vi "SMU Switch Handshaking - LV code improvements - Streaming.vi"(8 "error in":errorcluster, 9 "Error Stream gRPCid":T1, 10 "gRPCid":T1, 11 "file path (use dialog)":path=path "/home/lvuser/jsontestfile.json") -> (0 "error out":errorcluster, 3 "Elapsed Time":u32)   [LabVIEW 2019]
uses:
  VIs/MeasurementServer_gRPCid.ctl
  <instrlib>/niDCPower/nidcpower.llb/niDCPower Send Software Edge Trigger - Signal.ctl
  Global Operations.ctl
  VIs/MeasurementServer_FourProbeRawData.ctl
  VIs/MeasurementServer_ErrorOutData.ctl
  <instrlib>/niDCPower/nidcpower.llb/niDCPower Configure Software Edge Start Trigger.vi
  <instrlib>/niDCPower/nidcpower.llb/niDCPower Configure Software Edge Sequence Advance Trigger.vi
  VIs/labview-grpc-measurement-server.lvlib
  SupportVIs.lvlib
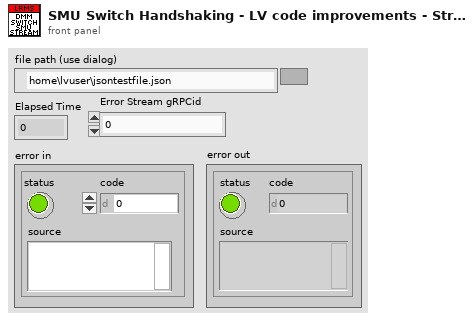
[diagram p1: front panel]
types:
  T1 = typedef "labview-grpc-measurement-server.lvlib/MeasurementServer_gRPCid.ctl" = u64
  T2 = typedef "niDCPower Send Software Edge Trigger - Signal.ctl" = i32
  T3 = typedef "JSONCluster.ctl" = cluster{"SMUResourceName":string, "SMUChannels":string, "SMUSourceMode":i32, "SMUOutputFunction":i32, "SMUSourceTransientResponse":i32, "SMUCurrent":dbl, "SMUCurrentLevelRange":dbl, "SMUMeasurementSense":i32, "SMUMeasurementApertureTime":dbl, "SMUSourceAdvancedSourceDelay":dbl, "SMUVoltage":dbl, "SMUSourceAdvancedSequenceLoopCount":i32, "SMUMeasurementAdvancedDCNoiseRejection":i32, "SMUSequenceName":string, "SMUStep1_Source_DCCurrent_CurrentLevel":i32, "SMUStep2_Measurement_ApertureTime":i32, "SMUStep3_Source_Advanced_SourceDelay":i32, "SMUSequenceNumberOfSteps":i32, "ScanList":string, "Switch1ResourceName":string, "Switch1Topology":string, "Switch1ScanList":string, "Switch2ResourceName":string, "Switch2Topology":string, "Switch2ScanList":string, "DMMResourceName":string, "DMMFunction":i32, "DMMResolution":dbl, "DMMRange":dbl, "DMMSampleCount":i32, "DMMApertureTimeUnit":i32, "DMMApertureTime":dbl, "DMMNumberOfAverages":i32, "DMMAutoZero":i32, "DMMADCCalibration":i32, "DMMSettleTime":dbl, "DMMControlAction":i32, "DMMVoltageFaultUpperLimit":dbl, "ApplicationNumberOfWeldChannels":i32}
  T4 = typedef "Global Operations.ctl" = enum16{"Get", "Set"}
  T5 = typedef "labview-grpc-measurement-server.lvlib/MeasurementServer_ErrorOutData.ctl" = cluster{"ErrorCode":i32, "ErrorMessage":string}
  T6 = typedef "labview-grpc-measurement-server.lvlib/MeasurementServer_FourProbeRawData.ctl" = cluster{"Positive Voltage":dbl, "Positive Current":dbl, "Negative Voltage":dbl, "Negative Current":dbl, "Impedance":dbl, "ErrorOutData":T5}
  T7 = typedef "niDMM Acquisition State.ctl" = enum16{"Running", "Finished with Backlog", "Finished with no Backlog", "Paused", "No acquisition in progress"}
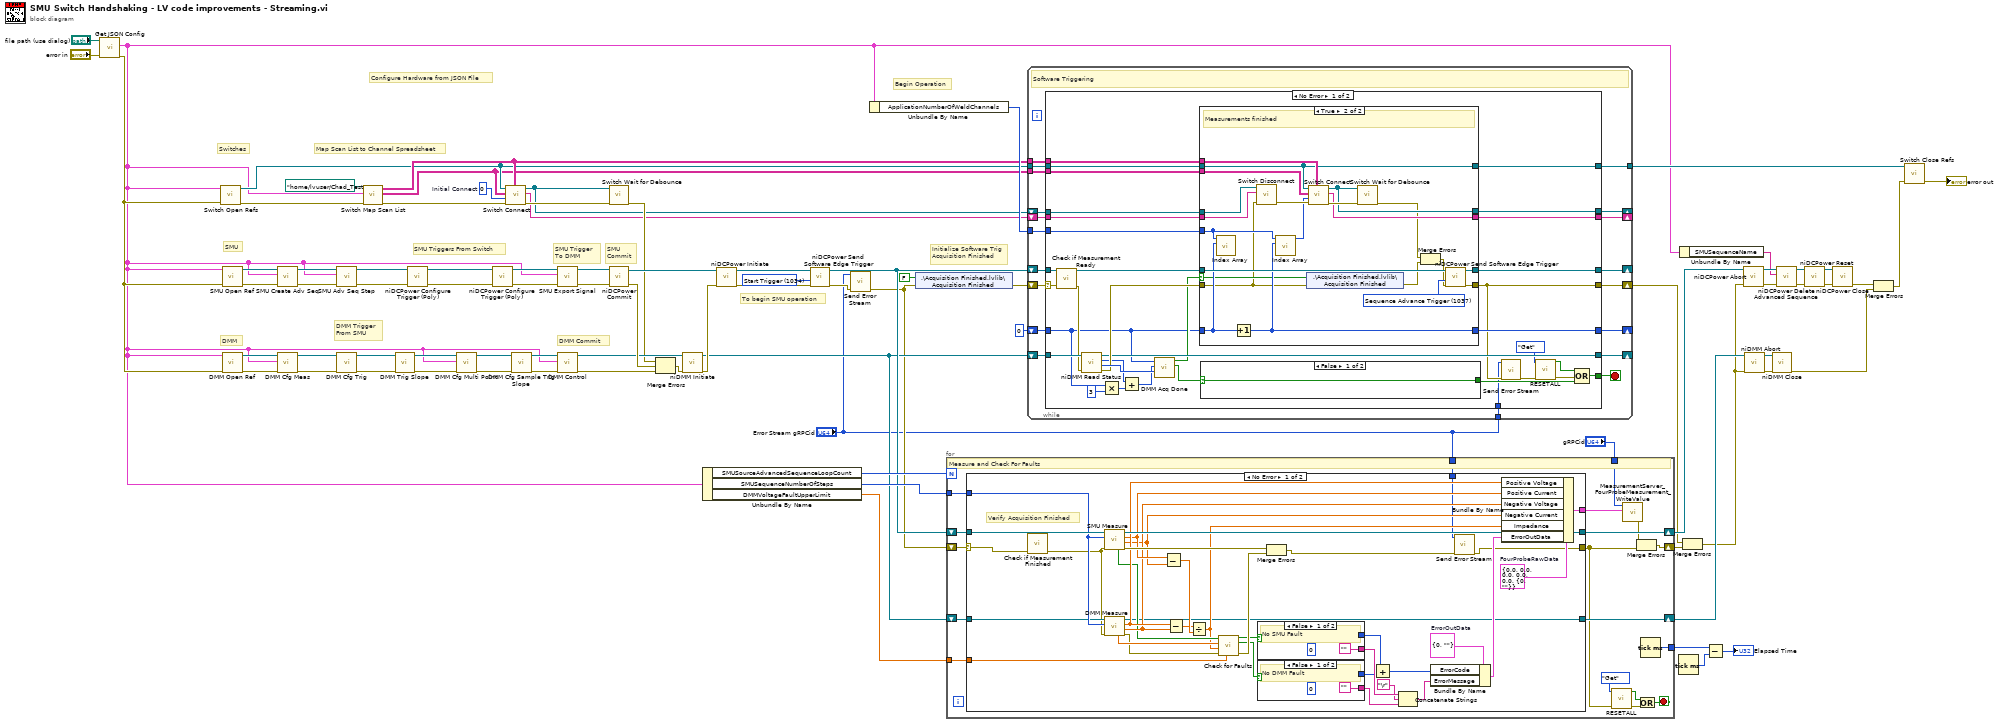
[diagram p0: block diagram]
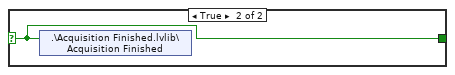
[diagram p2: hidden frame]
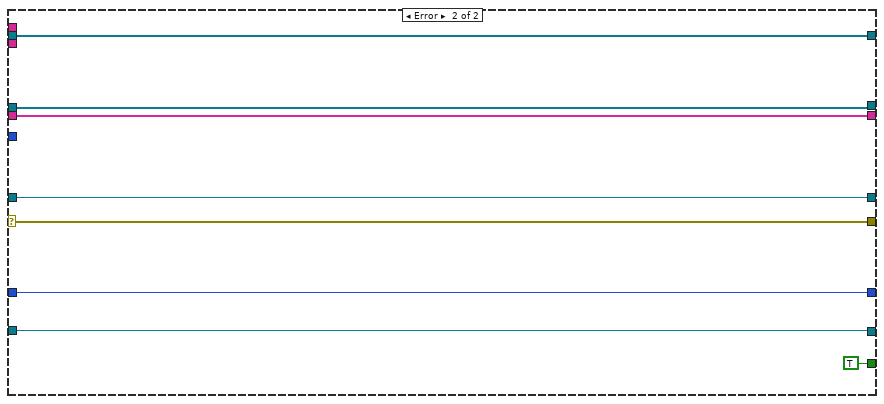
[diagram p4: hidden frame]
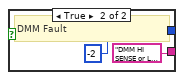
[diagram p5: hidden frame]
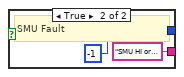
[diagram p6: hidden frame]
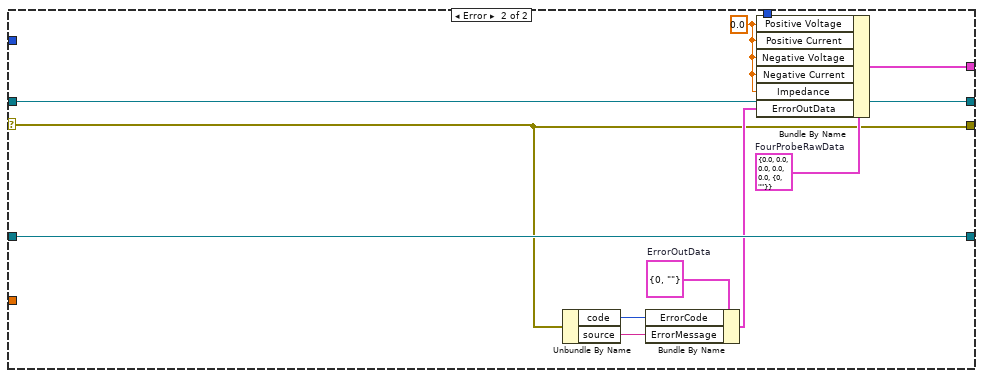
[diagram p7: hidden frame]
diagram:
  w12 = 0  # Initial Connect
  w35 = T2 1034 items=["Start Trigger"=1034, "Source Trigger"=1035, "Measure Trigger"=1036, "Sequence Advance Trigger"=1037, "Pulse Trigger"=1053] ("signal")
  # "Map Scan List to Channel Spreadsheet"
  # "Initialize Software Trig\nAcquisition Finished"
  # "SMU\nCommit"
  # "DMM Commit"
  # "Begin Operation"
  # "Configure Hardware from JSON File"
  # "DMM"
  # "SMU"
  # "Switches"
  # "To begin SMU operation"
  # "DMM Trigger\nFrom SMU"
  # "SMU Trigger \nTo DMM"
  # "SMU Triggers From Switch"
  n1 = call "Get JSON Config.vi"("error in (no error)"="error in", "JSON Configuration File (.json)"="file path (use dialog)") -> ("error out"=w11:errorcluster, "JSONCluster"=w1:T3)  [unwired: 6 in, 2 out]
  n2 = call "Switch Open Refs.vi"("error in (no error)"=w11, "JSONCluster"=w1) -> ("error out"=w15:errorcluster, "Switch Refs"=w8:refnum<k15>[])  [unwired: 8 in]
  n3 = call "SMU Open Ref.vi"("error in (no error)"=w11, "JSONCluster"=w1) -> ("error out"=w82:errorcluster, "IVI Refnum out"=w83:refnum<k15>)  [unwired: 8 in]
  n4 = call "DMM Open Ref.vi"("error in"=w11, "JSONCluster"=w1) -> ("error out"=w55:errorcluster, "IVI Refnum out"=w54:refnum<k15>)  [unwired: 8 in]
  n5 = call "SMU Create Adv Seq.vi"("error in (no error)"=w82, "JSONCluster"=w1, "IVI Refnum in"=w83) -> ("error out"=w70:errorcluster, "IVI Refnum out"=w71:refnum<k15>)  [unwired: 7 in]
  n6 = call "DMM Cfg Meas.vi"("error in (no error)"=w55, "JSONCluster"=w1, "IVI Refnum in"=w54) -> ("error out"=w59:errorcluster, "IVI Refnum out"=w58:refnum<k15>)  [unwired: 7 in]
  n7 = call "SMU Adv Seq Step.vi"("error in (no error)"=w70, "JSONCluster"=w1, "IVI Refnum in"=w71) -> ("error out"=w68:errorcluster, "IVI Refnum out"=w69:refnum<k15>)  [unwired: 7 in]
  n8 = call "DMM Cfg Trig.vi"("error in (no error)"=w59, "IVI Refnum in"=w58) -> ("error out"=w61:errorcluster, "IVI Refnum out"=w60:refnum<k15>)  [unwired: 8 in]
  n9 = call "Switch Map Scan List.vi"("error in (no error)"=w15, "JSONCluster"=w1, "Ch Spreadsheet"=path "/home/lvuser/Chad_Test.csv") -> ("error out"=w14:errorcluster, "IVI Specifications"=w7:string[][], "Channel Specs"=w9:string[][])  [unwired: 6 in]
  n10 = call "DMM Trig Slope.vi"("error in (no error)"=w61, "IVI Refnum in"=w60) -> ("error out"=w63:errorcluster, "IVI Refnum out"=w62:refnum<k15>)  [unwired: 8 in]
  n11 = call-poly <instrlib>:"niDCPower Configure Trigger (Poly).vi"("error in (no error)"=w68, "instrument handle"=w69) -> ("error out"=w79:errorcluster, "instrument handle out"=w80:refnum<k15>)  [unwired: 8 in]
  n12 = call "DMM Cfg Multi Point.vi"("error in (no error)"=w63, "JSONCluster"=w1, "IVI Refnum in"=w62) -> ("error out"=w65:errorcluster, "IVI Refnum out"=w64:refnum<k15>)  [unwired: 7 in]
  n13 = call-poly <instrlib>:"niDCPower Configure Trigger (Poly).vi"("error in (no error)"=w79, "instrument handle"=w80) -> ("error out"=w42:errorcluster, "instrument handle out"=w43:refnum<k15>)  [unwired: 8 in]
  n14 = call "Switch Connect.vi"("Channel Specs"=w9, "error in (no error)"=w14, "Channel Index"=w12, "IVI Specifications"=w7, "Switch Refs"=w8) -> ("error out"=w13:errorcluster, "Channels Connected"=w5:string[], "Refs Connected"=w6:refnum<k15>[])  [unwired: 4 in]
  n15 = call "DMM Cfg Sample Trig Slope.vi"("error in (no error)"=w65, "IVI Refnum in"=w64) -> ("error out"=w47:errorcluster, "IVI Refnum out"=w48:refnum<k15>)  [unwired: 8 in]
  n16 = call "SMU Export Signal.vi"("error in (no error)"=w42, "JSONCluster"=w1, "IVI Refnum in"=w43) -> ("error out"=w66:errorcluster, "IVI Refnum out"=w67:refnum<k15>)  [unwired: 7 in]
  n17 = call "DMM Control.vi"("error in (no error)"=w47, "JSONCluster"=w1, "IVI Refnum in"=w48) -> ("error out"=w52:errorcluster, "IVI Refnum out"=w49:refnum<k15>)  [unwired: 7 in]
  n18 = call "Switch Wait for Debounce.vi"("error in (no error)"=w13, "Switch Refs"=w6) -> ("error out"=w10:errorcluster)  [unwired: 9 in]
  n19 = call <instrlib>:"niDCPower Commit.vi"("error in (no error)"=w66, "instrument handle"=w67) -> ("error out"=w53:errorcluster, "instrument handle out"=w50:refnum<k15>)  [unwired: 8 in]
  n20 = Merge Errors(w10, w53, w52) -> (w51:errorcluster)
  n21 = call <instrlib>:"niDMM Initiate.vi"("error in (no error)"=w51, "instrument handle"=w49) -> ("error out"=w31:errorcluster, "instrument handle out"=w26:refnum<k15>)  [unwired: 8 in]
  n22 = Unbundle By Name(w1) -> ("SMUSourceAdvancedSequenceLoopCount"=w38:i32, "SMUSequenceNumberOfSteps"=w37:i32, "DMMVoltageFaultUpperLimit"=w22:dbl)
  n23 = call <instrlib>:"niDCPower Initiate.vi"("error in (no error)"=w31, "instrument handle"=w50) -> ("error out"=w32:errorcluster, "instrument handle out"=w36:refnum<k15>)  [unwired: 8 in]
  n24 = call <instrlib>:"niDCPower Send Software Edge Trigger.vi"("error in (no error)"=w32, "signal"=w35, "instrument handle"=w36) -> ("error out"=w19:errorcluster, "instrument handle out"=w27:refnum<k15>)  [unwired: 7 in]
  n25 = call "Send Error Stream.vi"("error in (no error)"=w19, "Error Stream gRPCid"="Error Stream gRPCid") -> ("error out"=w18:errorcluster)  [unwired: 9 in]
  n26 = Unbundle By Name(w1) -> ("ApplicationNumberOfWeldChannels"=w33:i32)
  n27 = shared-variable ".\\Acquisition Finished.lvlib\\Acquisition Finished"(FALSE ("Measurement Finished"), error in=w18) -> (error out=w24:errorcluster)
  n28 = for {
    N: w38 -> [_]
    tunnel: w37 -> [w96]
    shift-right: [w94] -> w28
    shift-left: w18 -> [w85]
    shift-right: [w101] -> w81
    shift-left: w27 -> [w97]
    shift-right: [w92] -> w44
    shift-left: w26 -> [w93]
    tunnel: [w100] -> w29
    tunnel: "gRPCid" -> [w99]
    tunnel: w22 -> [w91]
    tunnel: "Error Stream gRPCid" -> [w84]
    stop <- w86 stop-if-true
    # "Measure and Check For Faults"
    n29 = case shown="No Error" w85 {
      selector: w85 -> [w105 w147]
      tunnel: [w137 w155] -> w101
      tunnel: [w113 w148] -> w98
      tunnel: w97 -> [w112 w155]
      tunnel: w96 -> [w111 _]
      tunnel: w93 -> [w110 w154]
      tunnel: [w108 w154] -> w92
      tunnel: w91 -> [w106 _]
      tunnel: [w103 w147] -> w87
      tunnel: w84 -> [w102 _]
      frame No Error {
        w115 = T5 {"ErrorCode"=0, "ErrorMessage"=""}  # ErrorOutData
        w114 = T6 {"Positive Voltage"=0.0, "Positive Current"=0.0, "Negative Voltage"=0.0, "Negative Current"=0.0, "Impedance"=0.0, "ErrorOutData"={"ErrorCode"=0, "ErrorMessage"=""}}  # FourProbeRawData
        # "Verify Acquisition Finished"
        n30 = call "Check if Measurement Finished"("error in (no error)"=w105) -> ("error out"=w107:errorcluster)  [unwired: 10 in]
        n31 = call "SMU Measure.vi"("error in (no error)"=w107, "SMUSequenceNumberOfSteps"=w111, "IVI Refnum in"=w112) -> ("error out"=w136:errorcluster, "Numeric"=w129:dbl, "Numeric 2"=w131:dbl, "IVI Refnum out"=w137:refnum<k15>, "in compliance"=w118:bool[])  [unwired: 4 in]
        n32 = call "DMM Measure.vi"("error in (no error)"=w107, "SMUSequenceNumberOfSteps"=w111, "IVI Refnum in"=w110) -> ("error out"=w109:errorcluster, "Numeric"=w130:dbl, "Numeric 2"=w132:dbl, "IVI Refnum out"=w108:refnum<k15>, "Measurements"=w117:dbl[])  [unwired: 4 in]
        n33 = Subtract(x=w131, y=w129) -> (x-y=w134:dbl)
        n34 = Subtract(x=w132, y=w130) -> (x-y=w133:dbl)
        n35 = Divide(x=w133, y=w134) -> (x/y=w116:dbl)
        n36 = call "Check for Faults.vi"("DMM Voltage Fault Upper Limit"=w106, "Error In"=w109, "Resistance In"=w116, "dmm voltage measurements"=w117, "in compliance"=w118) -> ("Error Out"=w135:errorcluster, "DMM Fault"=w122:bool, "SMU Fault"=w126:bool)  [unwired: 3 in, 1 out]
        n37 = case shown="False" w126 {
          tunnel: ["" "SMU HI or LO lead disconnected\n- SMU in compliance\n- SMU Fault = True"] -> w125
          tunnel: [0 -1] -> w123
          frame False {
            # "No SMU Fault"
          }
          frame True {
            # "SMU Fault"
          }
        }
        n38 = case shown="False" w122 {
          tunnel: ["" "DMM HI SENSE or LO SENSE lead disconnected\n- DMM measures NaN, or \n- DMM overrange warning, or\n- DMM voltage > 50uV "] -> w120
          tunnel: [0 -2] -> w119
          frame False {
            # "No DMM Fault"
          }
          frame True {
            # "DMM Fault"
          }
        }
        n39 = Merge Errors(w136, w135) -> (w104:errorcluster)
        n40 = Add(x=w123, y=w119) -> (x+y=w127:i32)
        n41 = Concatenate Strings(w125, "\r", w120) -> (w124:string)
        n42 = Bundle By Name(cluster=w115, "ErrorCode"=w127, "ErrorMessage"=w124) -> (w128:T5)
        n43 = call "Send Error Stream.vi"("error in (no error)"=w104, "Error Stream gRPCid"=w102) -> ("error out"=w103:errorcluster)  [unwired: 9 in]
        n44 = Bundle By Name(cluster=w114, "Positive Voltage"=w132, "Positive Current"=w131, "Negative Voltage"=w130, "Negative Current"=w129, "Impedance"=w116, "ErrorOutData"=w128) -> (w113:T6)
      }
      frame Error {
        w146 = 0.0 ("Positive Voltage")
        w151 = T5 {"ErrorCode"=0, "ErrorMessage"=""}  # ErrorOutData
        w152 = T6 {"Positive Voltage"=0.0, "Positive Current"=0.0, "Negative Voltage"=0.0, "Negative Current"=0.0, "Impedance"=0.0, "ErrorOutData"={"ErrorCode"=0, "ErrorMessage"=""}}  # FourProbeRawData
        n45 = Unbundle By Name(w147) -> ("code"=w149:i32, "source"=w150:string)
        n46 = Bundle By Name(cluster=w151, "ErrorCode"=w149, "ErrorMessage"=w150) -> (w153:T5)
        n47 = Bundle By Name(cluster=w152, "Positive Voltage"=w146, "Positive Current"=w146, "Negative Voltage"=w146, "Negative Current"=w146, "Impedance"=w146, "ErrorOutData"=w153) -> (w148:T6)
      }
    }
    n48 = call "RESETALL.vi"("error in (no error)"=w87, "Operation"=Global_Operations."Get") -> ("error out"=w89:errorcluster, "RESETALL?"=w88:bool)  [unwired: 8 in]
    n49 = call "MeasurementServer_FourProbeMeasurement_WriteValue.vi"("gRPCid"=w99, "FourProbeRawData"=w98) -> ("error out"=w95:errorcluster)  [unwired: 8 in]
    n50 = Merge Errors(w95, w87) -> (w94:errorcluster)
    n51 = Compound Arithmetic op=OR(w88, w89) -> (w86:bool)
    n52 = Tick Count (ms)() -> (millisecond timer value=w100:u32)
  }
  n53 = while {
    shift-right: [w174] -> _
    shift-left: w27 -> [w173]
    shift-right: [w167] -> w25
    shift-left: w24 -> [w165]
    shift-right: [w169] -> _
    shift-left: w26 -> [w170]
    shift-right: [w172] -> _
    shift-left: 0 ("Backlog") -> [w168]
    tunnel: w33 -> [w171]
    tunnel: "Error Stream gRPCid" -> [w164]
    tunnel: w9 -> [w163]
    tunnel: w8 -> [w162]
    tunnel: w7 -> [w161]
    shift-right: [w157] -> _
    shift-left: w6 -> [w160]
    shift-right: [w156] -> _
    shift-left: w5 -> [w159]
    tunnel: [w158] -> w4
    stop <- w166 stop-if-true
    # "Software Triggering"
    n54 = case shown="No Error" w165 {
      selector: w165 -> [w186 w242]
      tunnel: [w207 w241] -> w174
      tunnel: w173 -> [w206 w241]
      tunnel: [w205 w243] -> w172
      tunnel: w171 -> [w204 _]
      tunnel: w170 -> [w202 w244]
      tunnel: [w200 w244] -> w169
      tunnel: w168 -> [w195 w243]
      tunnel: [w185 w242] -> w167
      tunnel: [w187 TRUE] -> w166
      tunnel: w164 -> [w183 _]
      tunnel: w163 -> [w182 _]
      tunnel: w162 -> [w181 w240]
      tunnel: w161 -> [w180 _]
      tunnel: w160 -> [w179 w239]
      tunnel: w159 -> [w178 w238]
      tunnel: [w177 w240] -> w158
      tunnel: [w176 w239] -> w157
      tunnel: [w175 w238] -> w156
      frame No Error {
        n55 = call "Check if Measurement Ready.vi"("error in (no error)"=w186) -> ("error out"=w198:errorcluster)  [unwired: 10 in]
        n56 = call <instrlib>:"niDMM Read Status.vi"("error in (no error)"=w198, "instrument handle"=w202) -> ("error out"=w201:errorcluster, "Acquisition State"=w203:T7, "Backlog"=w197:i32, "instrument handle out"=w200:refnum<k15>)  [unwired: 6 in]
        n57 = Multiply(x=w195, y=3) -> (x*y=w193:i32)
        n58 = Add(x=w197, y=w193) -> (x+y=w196:i32)
        n59 = call "DMM Acq Done.vi"("Acquisition State"=w203, "Backlog"=w196, "Channel Index"=w195) -> ("Finished with Backlog?"=w192:bool, "Sequence Acquision Finished?"=w199:bool)  [unwired: 7 in]
        n60 = case shown="True" w199 {
          selector: w199 -> [_ w229]
          tunnel: w201 -> [w214 w216]
          tunnel: [w215 w237] -> w207
          tunnel: [w214 w236] -> w185
          tunnel: w206 -> [w215 w234]
          tunnel: w195 -> [w213 w232]
          tunnel: [w213 w231] -> w205
          tunnel: w204 -> [_ w230]
          tunnel: w182 -> [_ w225]
          tunnel: w181 -> [w212 w220]
          tunnel: w180 -> [_ w224]
          tunnel: w179 -> [w211 w223]
          tunnel: w178 -> [w210 w222]
          tunnel: [w212 w220] -> w177
          tunnel: [w211 w219] -> w176
          tunnel: [w210 w218] -> w175
          frame False {
            # "Measurements not finished yet - repeat loop"
          }
          frame True {
            w235 = T2 1037 items=["Start Trigger"=1034, "Source Trigger"=1035, "Measure Trigger"=1036, "Sequence Advance Trigger"=1037, "Pulse Trigger"=1053] ("signal")
            # "Measurements finished"
            n61 = call "Index Array.vi"("Backlog"=w232, "ApplicationNumberOfWeldChannels"=w230) -> ()  [unwired: 9 in, 1 out]
            n62 = Increment(x=w232) -> (x+1=w231:i32)
            n63 = call "Switch Disconnect.vi"("error in (no error)"=w216, "Channels Connected"=w222, "Switch Refs"=w223) -> ("error out"=w227:errorcluster)  [unwired: 8 in]
            n64 = call "Index Array.vi"("Backlog"=w231, "ApplicationNumberOfWeldChannels"=w230) -> ("Index"=w221:i32)  [unwired: 9 in]
            n65 = shared-variable ".\\Acquisition Finished.lvlib\\Acquisition Finished"(w229, error in=w216) -> (error out=w228:errorcluster)
            n66 = call "Switch Connect.vi"("Channel Specs"=w225, "error in (no error)"=w227, "Channel Index"=w221, "IVI Specifications"=w224, "Switch Refs"=w220) -> ("error out"=w226:errorcluster, "Channels Connected"=w218:string[], "Refs Connected"=w219:refnum<k15>[])  [unwired: 4 in]
            n67 = call "Switch Wait for Debounce.vi"("error in (no error)"=w226, "Switch Refs"=w219) -> ("error out"=w217:errorcluster)  [unwired: 9 in]
            n68 = Merge Errors(w217, w228) -> (w233:errorcluster)
            n69 = call <instrlib>:"niDCPower Send Software Edge Trigger.vi"("error in (no error)"=w233, "signal"=w235, "instrument handle"=w234) -> ("error out"=w236:errorcluster, "instrument handle out"=w237:refnum<k15>)  [unwired: 7 in]
          }
        }
        n70 = case shown="False" w192 {
          selector: w192 -> [w208 w209]
          tunnel: [w208 w209] -> w188
          frame False {
          }
          frame True {
            n71 = shared-variable ".\\Acquisition Finished.lvlib\\Acquisition Finished"(w209) -> ()  [unwired: 1 in, 1 out]
          }
        }
        n72 = call "Send Error Stream.vi"("error in (no error)"=w185, "Error Stream gRPCid"=w183) -> ("error out"=w184:errorcluster)  [unwired: 9 in]
        n73 = call "RESETALL.vi"("error in (no error)"=w184, "Operation"=Global_Operations."Get") -> ("error out"=w190:errorcluster, "RESETALL?"=w189:bool)  [unwired: 8 in]
        n74 = Compound Arithmetic op=OR(w189, w190, w188) -> (w187:bool)
      }
      frame Error {
      }
    }
  }
  n75 = Tick Count (ms)() -> (millisecond timer value=w78:u32)
  n76 = Unbundle By Name(w1) -> ("SMUSequenceName"=w30:string)
  n77 = Merge Errors(w25, w28) -> (w20:errorcluster)
  n78 = Subtract(x=w29, y=w78) -> (x-y=→"Elapsed Time":u32)
  n79 = call <instrlib>:"niDCPower Abort.vi"("error in (no error)"=w20, "instrument handle"=w81) -> ("error out"=w76:errorcluster, "instrument handle out"=w77:refnum<k15>)  [unwired: 8 in]
  n80 = call <instrlib>:"niDMM Abort.vi"("error in (no error)"=w20, "instrument handle"=w44) -> ("error out"=w57:errorcluster, "instrument handle out"=w56:refnum<k15>)  [unwired: 8 in]
  n81 = call <instrlib>:"niDMM Close.vi"("error in (no error)"=w57, "instrument handle"=w56) -> ("error out"=w46:errorcluster)  [unwired: 9 in]
  n82 = call <instrlib>:"niDCPower Delete Advanced Sequence.vi"("error in (no error)"=w76, "sequence name"=w30, "instrument handle"=w77) -> ("error out"=w75:errorcluster, "instrument handle out"=w74:refnum<k15>)  [unwired: 7 in]
  n83 = call <instrlib>:"niDCPower Reset.vi"("error in (no error)"=w75, "instrument handle"=w74) -> ("error out"=w72:errorcluster, "instrument handle out"=w73:refnum<k15>)  [unwired: 2 in, 6 out]
  n84 = call <instrlib>:"niDCPower Close.vi"("error in (no error)"=w72, "instrument handle"=w73) -> ("error out"=w45:errorcluster)  [unwired: 9 in]
  n85 = Merge Errors(w45, w46) -> (w3:errorcluster)
  n86 = call "Switch Close Refs.vi"("error in (no error)"=w3, "Switch Refs"=w4) -> ("error out"=→"error out":errorcluster)  [unwired: 9 in]
